vi "Keithley2400series_Relay_2_set Ch.vi"(6 "Ch4":bool, 7 "Ch1":bool, 8 "error in (no error)":errorcluster, 9 "Ch3":bool, 10 "Ch2":bool, 11 "VISA Refnum in":refnum<visa-resource-name>) -> (0 "error out":errorcluster, 3 "VISA Refnum out":refnum<visa-resource-name>)   [LabVIEW 2014]
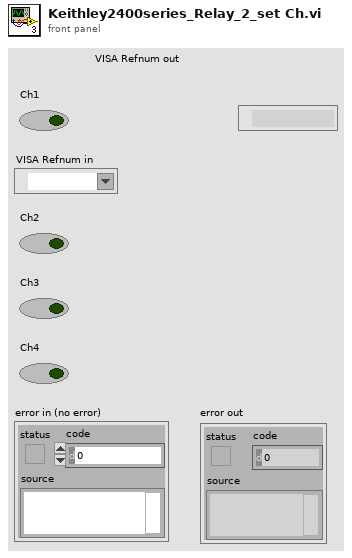
[diagram p1: front panel]
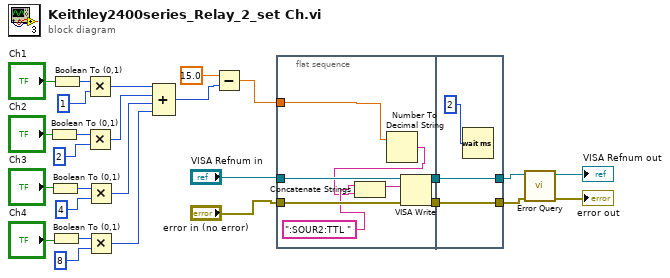
[diagram p0: block diagram]
diagram:
  n1 = Boolean To (0,1)(Boolean="Ch2") -> (0, 1=w7:i16)
  n2 = Boolean To (0,1)(Boolean="Ch3") -> (0, 1=w8:i16)
  n3 = Boolean To (0,1)(Boolean="Ch4") -> (0, 1=w9:i16)
  n4 = Boolean To (0,1)(Boolean="Ch1") -> (0, 1=w6:i16)
  n5 = Multiply(x=w6, y=i16 1) -> (x*y=w14:i16)
  n6 = Multiply(x=w7, y=i16 2) -> (x*y=w15:i16)
  n7 = Multiply(x=w8, y=i16 4) -> (x*y=w16:i16)
  n8 = Multiply(x=w9, y=i16 8) -> (x*y=w17:i16)
  n9 = Compound Arithmetic op=ADD(w14, w15, w16, w17) -> (w19:i16)
  n10 = Subtract(x=15.0, y=w19) -> (x-y=w23:dbl)
  n11 = flat-sequence {
    tunnel: [w35] -> w27
    tunnel: [w34] -> w26
    tunnel: "VISA Refnum in" -> [w33]
    tunnel: "error in (no error)" -> [w32]
    tunnel: w23 -> [w28]
    tunnel: [w37] -> w25
    tunnel: [w38] -> w24
    tunnel: w27 -> [w38]
    tunnel: w26 -> [w37]
    frame #0 {
      n12 = Number To Decimal String(number=w28) -> (decimal integer string=w29:string)  [unwired: 1 in]
      n13 = Concatenate Strings(":SOUR2:TTL " ("string"), w29) -> (w31:string)
      n14 = VISA Write(VISA resource name=w33, write buffer=w31, error in (no error)=w32) -> (VISA resource name out=w35:refnum<visa-resource-name>, error out=w34:errorcluster)  [unwired: 1 out]
    }
    frame #1 {
      n15 = Wait (ms)(milliseconds to wait=u32 2) -> ()  [unwired: 1 out]
    }
  }
  n16 = call "Error Query.vi"("error in (no error)"=w25, "VISA resource name"=w24) -> ("error out"=→"error out":errorcluster, "VISA resource name out"=→"VISA Refnum out":refnum<visa-resource-name>)  [unwired: 6 in, 2 out]
